vi "ExtendedRegisterRead_No hardware compare.vi"(7 "Extended Read/Write":T1 {"Data" format="%.0x"; "Register" format="%.0x"; "Slave Address" max=15 format="%.0x"}, 8 "error in (no error)":errorcluster, 9 "Number of Samples In":i32, 10 "Data Array":u8[][](array[numeric]), 11 "RFFE_Data In":T2 {"Toggle (high to low)" items=["0", "1", "Z", "L", "H", "X", "T", "V"]; "X Array" items=["0", "1", "Z", "L", "H", "X", "T", "V"]; "Z Array" items=["0", "1", "Z", "L", "H", "X", "T", "V"]; "L Array" items=["0", "1", "Z", "L", "H", "X", "T", "V"]; "H Array" items=["0", "1", "Z", "L", "H", "X", "T", "V"]; "One Array" items=["0", "1", "Z", "L", "H", "X", "T", "V"]; "Zero Array" items=["0", "1", "Z", "L", "H", "X", "T", "V"]}) -> (0 "error out":errorcluster, 1 "Number of Samples Out out":i32, 2 "Data Array Out":u8[][](array[numeric]), 3 "RFFE_Data Out":T2 {"Toggle (high to low)" items=["0", "1", "Z", "L", "H", "X", "T", "V"]; "X Array" items=["0", "1", "Z", "L", "H", "X", "T", "V"]; "Z Array" items=["0", "1", "Z", "L", "H", "X", "T", "V"]; "L Array" items=["0", "1", "Z", "L", "H", "X", "T", "V"]; "H Array" items=["0", "1", "Z", "L", "H", "X", "T", "V"]; "One Array" items=["0", "1", "Z", "L", "H", "X", "T", "V"]; "Zero Array" items=["0", "1", "Z", "L", "H", "X", "T", "V"]})   [LabVIEW 2013]
doc: "Builds MIPI RFFE Extended Register Read with the specified data."
uses:
  Ctrls/RFFE_Data.ctl
  Ctrls/ClockDataChannels.ctl
  Ctrls/ExtendedRegReadWrite.ctl
  Ctrls/Commands.ctl
  Ctrls/Read_Write_Data.ctl
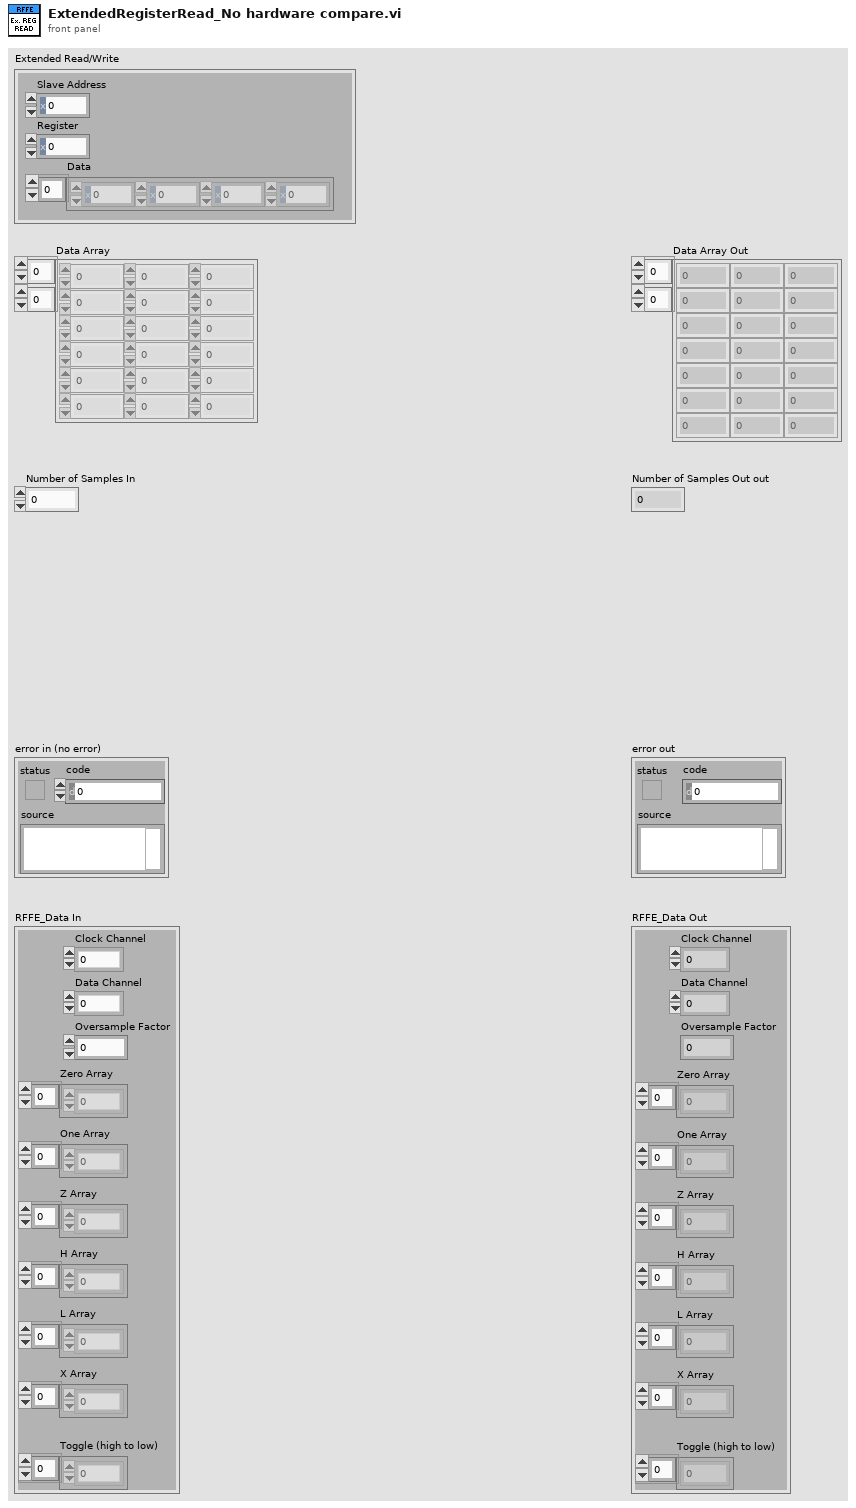
[diagram p1: front panel]
types:
  T1 = typedef "ExtendedRegReadWrite.ctl" = cluster{"Slave Address":u8, "Register":u8, "Data":u8[]}
  T2 = typedef "RFFE_Data.ctl" = cluster{"Clock Channel":T3, "Data Channel":T3, "Oversample Factor":u8, "Zero Array":u8[], "One Array":u8[], "Z Array ":u8[], "H Array":u8[], "L Array":u8[], "X Array":u8[], "Toggle (high to low)":u8[]}
  T3 = typedef "ClockDataChannels.ctl" = enum16{"0", "1"}
  T4 = typedef "Read_Write_Data.ctl" = cluster{"Data":u8, "Read/Write":enum16{"Read", "Write"}}
  T5 = typedef "Commands.ctl" = cluster{"Command":enum16{"Extended Register Write", "Extended Register Read", "Extended Register Write Long", "Extended Register Read Long", "Register Write", "Register Read", "Register 0 Write"}, "Data/Address/ByteCount":u8}
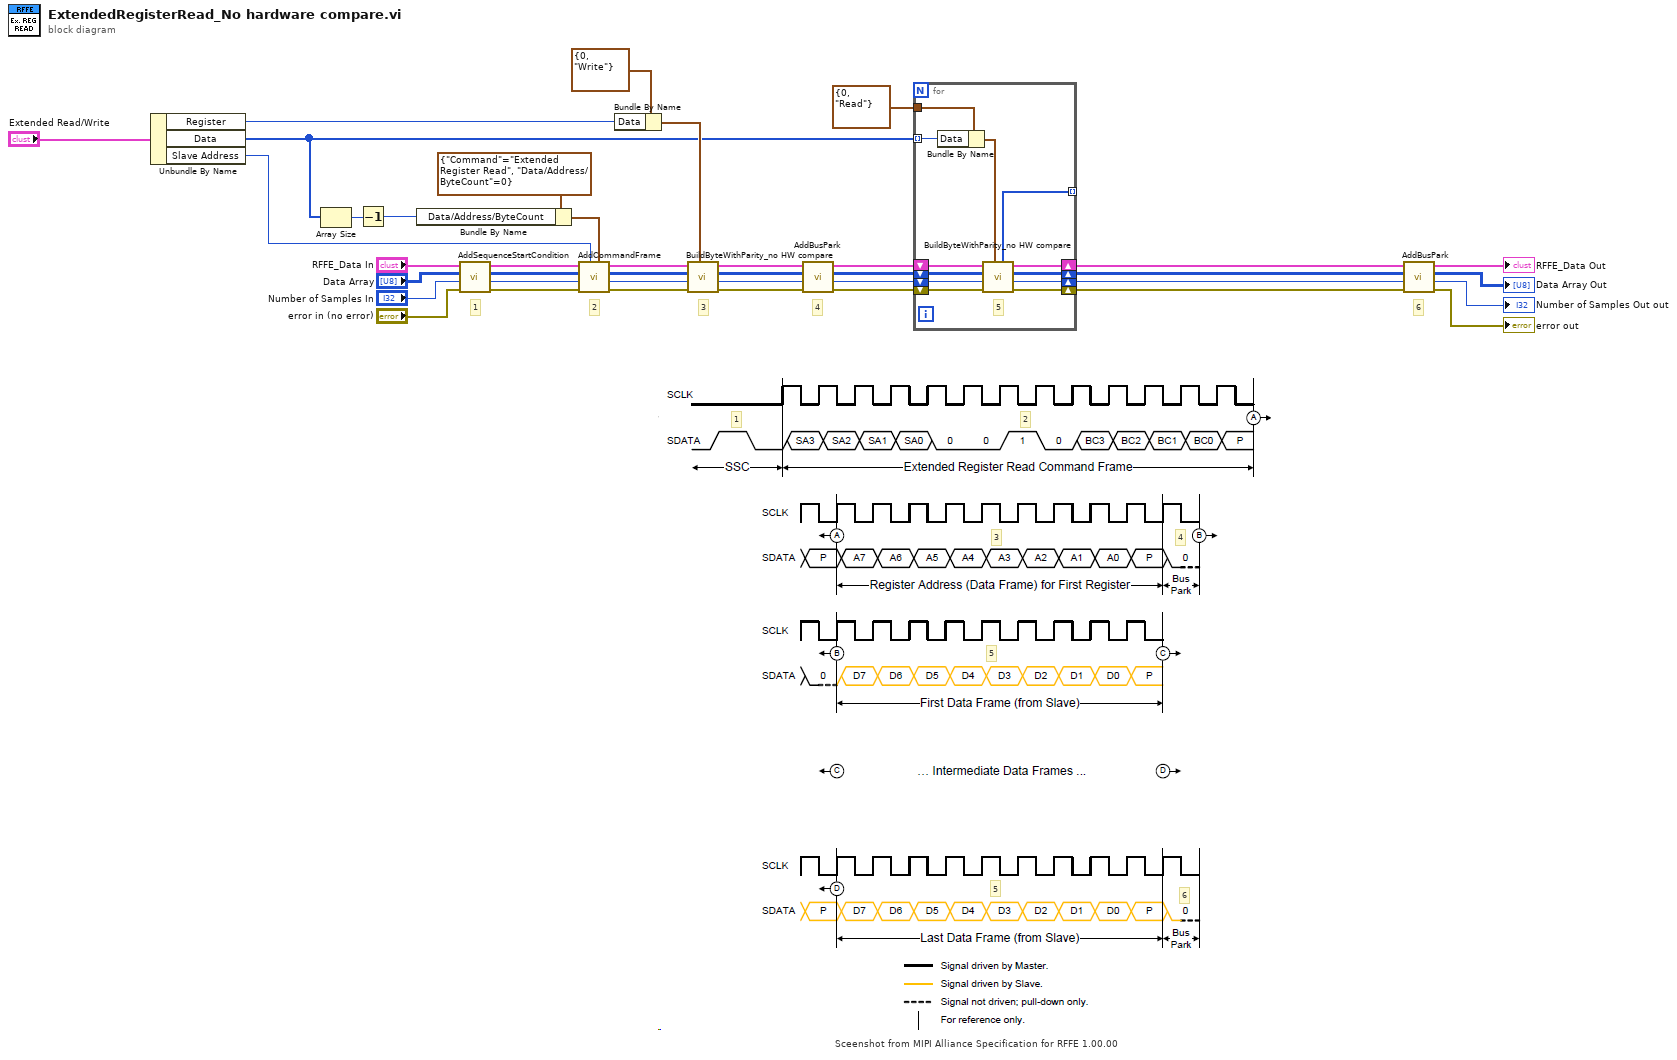
[diagram p0: block diagram]
diagram:
  # "5"
  # "Sceenshot from MIPI Alliance Specification for RFFE 1.00.00"
  # "6"
  # "5"
  # "4"
  # "3"
  # "2"
  # "1"
  # "6"
  # "4"
  # "3"
  # "2"
  # "1"
  n1 = Unbundle By Name("Extended Read/Write") -> ("Register"=w4:u8, "Data"=w3:u8[], "Slave Address"=w8:u8)
  n2 = Array Size(array=w3) -> (size(s)=w21:i32)
  n3 = Decrement(x=w21) -> (x-1=w18:i32)
  n4 = Bundle By Name(cluster=T5 {"Command"=enum."Extended Register Read", "Data/Address/ByteCount"=0} ("Command"), "Data/Address/ByteCount"=w18) -> (w9:T5)
  n5 = call "AddSequenceStartCondition.vi"("error in (no error)"="error in (no error)", "Number of Samples In"="Number of Samples In", "Data Array In"="Data Array", "RFFE_Data In"="RFFE_Data In") -> ("error out"=w31:errorcluster, "Number of Samples Out"=w37:i32, "Data Array Out"=w32:u8[][], "RFFE_Data Out"=w33:T2)  [unwired: 4 in]
  n6 = call "AddCommandFrame.vi"("Command"=w9, "Slave Address"=w8, "error in (no error)"=w31, "Number of Samples In"=w37, "Data Array In"=w32, "RFFE_Data"=w33) -> ("error out"=w34:errorcluster, "Number of Samples Out"=w10:i32, "Data Array Out"=w11:u8[][], "Configuratation Out"=w35:T2)  [unwired: 2 in]
  n7 = Bundle By Name(cluster=T4 {"Data"=0, "Read/Write"=enum."Write"} ("Read/Write Data"), "Data"=w4) -> (w19:T4)
  n8 = call "BuildByteWithParity_no HW compare.vi"("Read/Write Data"=w19, "error in"=w34, "Number of Samples In"=w10, "Data Array In"=w11, "RFFE_Data In"=w35) -> ("error out"=w14:errorcluster, "Number of Samples Out"=w12:i32, "Data Array Out"=w13:u8[][], "RFFE_Data Out"=w15:T2)  [unwired: 2 in, 1 out]
  n9 = call "AddBusPark.vi"("error in (no error)"=w14, "Number of Samples In"=w12, "Data Array In"=w13, "RFFE_Data In"=w15) -> ("error out"=w16:errorcluster, "Number of Samples Out"=w5:i32, "Data Array Out"=w6:u8[][], "RFFE_Data Out"=w7:T2)  [unwired: 4 in]
  n10 = for {
    shift-right: [w50] -> w24
    shift-left: w16 -> [w51]
    shift-right: [w47] -> w22
    shift-left: w5 -> [w49]
    shift-right: [w46] -> w23
    shift-left: w6 -> [w48]
    shift-right: [w45] -> w2
    shift-left: w7 -> [w44]
    tunnel: w3 -> [w40] mode=indexing
    tunnel: T4 {"Data"=0, "Read/Write"=enum."Read"} ("Read/Write Data") -> [w42]
    tunnel: [w41] -> _ mode=indexing
    # "5"
    n11 = Bundle By Name(cluster=w42, "Data"=w40) -> (w43:T4)
    n12 = call "BuildByteWithParity_no HW compare.vi"("Read/Write Data"=w43, "error in"=w51, "Number of Samples In"=w49, "Data Array In"=w48, "RFFE_Data In"=w44) -> ("error out"=w50:errorcluster, "Number of Samples Out"=w47:i32, "Data Array Out"=w46:u8[][], "RFFE_Data Out"=w45:T2, "Compare Locations"=w41:u32[])  [unwired: 2 in]
  }
  n13 = call "AddBusPark.vi"("error in (no error)"=w24, "Number of Samples In"=w22, "Data Array In"=w23, "RFFE_Data In"=w2) -> ("error out"=→"error out":errorcluster, "Number of Samples Out"=→"Number of Samples Out out":i32, "Data Array Out"=→"Data Array Out":u8[][], "RFFE_Data Out"=→"RFFE_Data Out":T2)  [unwired: 4 in]
